vi "Build Client Table.vi"(8 "error in (no error)":errorcluster, 11 "System Status Module in":refnum<class "System Status Module.lvclass">) -> (0 "error out":errorcluster, 2 "Clients":T1[](array[typedef]), 3 "System Status Module out":refnum<class "System Status Module.lvclass">)   [LabVIEW 2020, in "VolatusGUI.lvlib" / "System Status Module.lvclass"]
uses:
  System Status Module.lvclass
  C:/dev/lv20CE/relink/lv-volatus/Volatus/Module/Module.lvclass
  Client Row.ctl
  Volatus/Module/Module.lvclass/Module.ctl
  System Status Module.lvclass/System Status Module.ctl
  Volatus/Module/Module.lvclass
  Volatus/VolatusAPI/VolatusAPI.lvclass
  VolatusConfig/VolatusConfig/VolatusConfig.lvclass
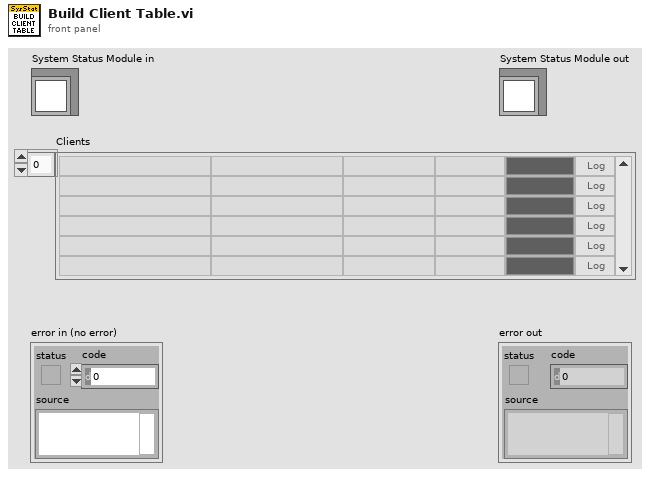
[diagram p1: front panel]
types:
  T1 = typedef "VolatusGUI.lvlib/System Status Module.lvclass/Client Row.ctl" = cluster{"Node":string, "Alias":string, "IP":string, "App Version":string, "Cfg Version":string, "Debug Log":bool, "Cfg Color":u32}
  T2 = typedef "TcpClientList.lvlib/Data.ctl" = cluster{"clients":T3[]}
  T3 = typedef "TcpClientInfo.lvlib/Data.ctl" = cluster{"node_id":u32, "node_name":string, "app_version":string, "config_version":string, "config_hash":string, "node_alias":string, "address":string}
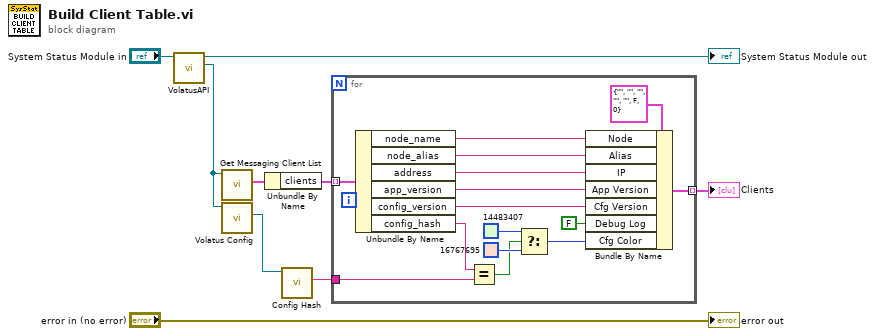
[diagram p0: block diagram]
diagram:
  n1 = call "VolatusAPI.vi"("Module in"="System Status Module in") -> ("VolatusAPI"=w3:refnum<class "VolatusAPI.lvclass">, "Module out"=→"System Status Module out":refnum<class "System Status Module.lvclass">)  [unwired: 9 in]
  n2 = call "Get Messaging Client List.vi"("VolatusAPI in"=w3) -> ("Client List"=w6:T2)  [unwired: 8 in, 2 out]
  n3 = call "Volatus Config.vi"("VolatusAPI in"=w3) -> ("Volatus Config"=w2:refnum<class "VolatusConfig.lvclass">)  [unwired: 8 in, 2 out]
  n4 = Unbundle By Name(w6) -> ("clients"=w5:T3[])
  n5 = call "Config Hash.vi"("VolatusConfig in"=w2) -> ("Config Hash"=w1:string)  [unwired: 8 in, 2 out]
  n6 = for {
    tunnel: w5 -> [w24] mode=indexing
    tunnel: [w16] -> w4 mode=indexing
    tunnel: w1 -> [w12]
    n7 = Unbundle By Name(w24) -> ("node_name"=w22:string, "node_alias"=w21:string, "address"=w20:string, "app_version"=w19:string, "config_version"=w18:string, "config_hash"=w13:string)
    n8 = Equal?(x=w13, y=w12) -> (x = y?=w11:bool)
    n9 = Select(t=u32 14483407, s=w11, f=u32 16767695) -> (s? t:f=w10:u32)
    n10 = Bundle By Name(cluster=T1 {"Node"="", "Alias"="", "IP"="", "App Version"="", "Cfg Version"="", "Debug Log"=FALSE, "Cfg Color"=0} ("Client Row"), "Node"=w22, "Alias"=w21, "IP"=w20, "App Version"=w19, "Cfg Version"=w18, "Debug Log"=FALSE, "Cfg Color"=w10) -> (w16:T1)
  }
  "Clients" <- w4
  "error out" <- "error in (no error)"
